vi "Configure Power Measurement Parameter Bandwidth.vi"(6 "Bandwidth":dbl[](array[numeric]) format="%#.9p", 7 "Filter Type (Gauss)":i32(ring) items=["Gauss", "Bandpass"], 8 "error in (no error)":errorcluster, 9 "Array Size (32)":i32=32, 10 "Instance (1)":i32=1, 11 "VISA resource name":refnum<visa-resource-name>) -> (0 "error out":errorcluster, 3 "VISA resource name out":refnum<visa-resource-name>)   [LabVIEW 2020, in "Rohde&Schwarz CMXP GPRF.lvlib"]
doc: "This VI sets is a combination of measurement control settings. The \"Parameter Set List\" contains 32 possibly different parameter sets which you may assign to the individual measurement steps in list mode.\n\nAttributes:\nRSCMXPGPRF_ATTR_POWER_MEASUREMENT_PARAMETER_SET_GAUSS_BW_ALL\nRSCMXPGPRF_ATTR_POWER_MEASUREMENT_PARAMETER_SET_BANDPASS_BW_ALL\n\nRemote-control commands:\nCONFigure:GPRF:MEAS<i>:POWer:PSET:FILTer:GAUSs:BWIDth:ALL\nCONFigure:GPRF:MEAS<i>:POWer:PSET:FILTer:BANDpass:BWIDth:ALL"
uses:
  <instrlib>/Rohde&Schwarz CMXP GPRF/Rohde&Schwarz CMXP GPRF.lvlib
  <instrlib>/Rohde&Schwarz CMXP GPRF/Private/rsidr_core.llb/rsidr_core.lvlib
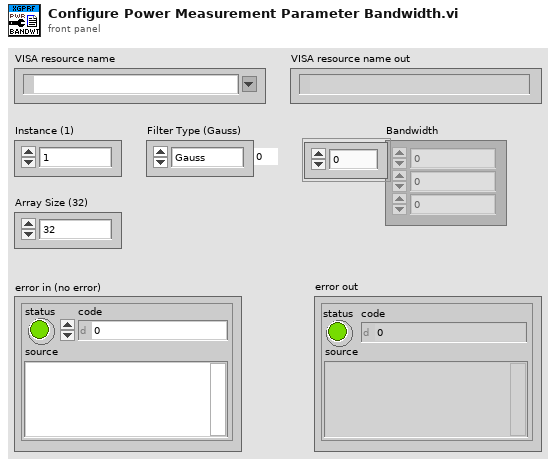
[diagram p1: front panel]
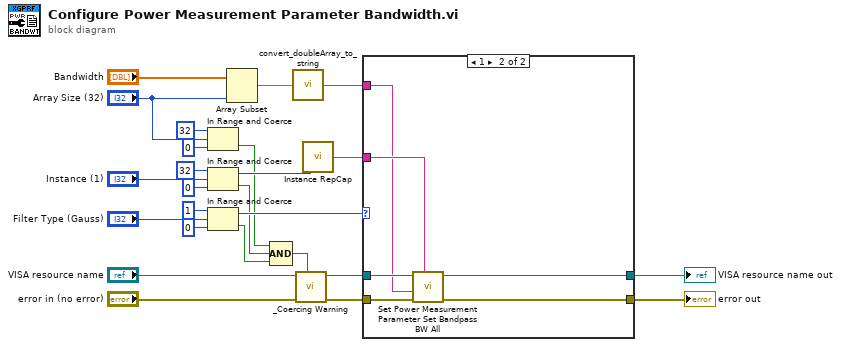
[diagram p0: block diagram]
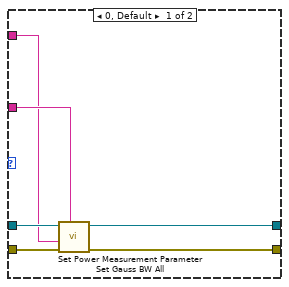
[diagram p2: hidden frame]
diagram:
  n1 = In Range and Coerce(upper limit=32, x="Array Size (32)", lower limit=0) -> (In Range?=w1:bool)  [unwired: 1 out]
  n2 = In Range and Coerce(upper limit=32, x="Instance (1)", lower limit=0) -> (coerced(x)=w14:i32, In Range?=w2:bool)
  n3 = In Range and Coerce(upper limit=1, x="Filter Type (Gauss)", lower limit=0) -> (coerced(x)=w10:i32, In Range?=w3:bool)
  n4 = Array Subset(array="Bandwidth", length="Array Size (32)") -> (w18:dbl[])  [unwired: 1 in]
  n5 = Compound Arithmetic op=AND(w1, w2, w3) -> (w21:bool)
  n6 = call <instrlib>:"convert_doubleArray_to_string.vi"("double array in"=w18) -> ("string out"=w4:string)  [unwired: 4 in]
  n7 = call <instrlib>:"_Coercing Warning.vi"("In Range?"=w21, "error in (no error)"="error in (no error)", "VISA resource name"="VISA resource name") -> ("error out"=w9:errorcluster, "VISA resource name out"=w8:refnum<visa-resource-name>)  [unwired: 7 in]
  n8 = call <instrlib>:"Instance RepCap.vi"("Instance in"=w14) -> ("Instance out"=w5:string)
  n9 = case shown="1" w10 {
    tunnel: w9 -> [w31 w37]
    tunnel: w8 -> [w30 w36]
    tunnel: [w29 w35] -> w7
    tunnel: [w28 w34] -> w6
    tunnel: w5 -> [w27 w33]
    tunnel: w4 -> [w26 w32]
    frame 0, Default {
      n10 = call "Set Power Measurement Parameter Set Gauss BW All"("Repeated Capabilities"=w27, "error in (no error)"=w31, "Power Measurement Parameter Set Gauss BW All ()"=w26, "instrument handle"=w30) -> ("error out"=w29:errorcluster, "instrument handle out"=w28:refnum<visa-resource-name>)  [unwired: 6 in]
    }
    frame 1 {
      n11 = call "Set Power Measurement Parameter Set Bandpass BW All"("Repeated Capabilities"=w33, "error in (no error)"=w37, "Power Measurement Parameter Set Bandpass BW All ()"=w32, "instrument handle"=w36) -> ("error out"=w35:errorcluster, "instrument handle out"=w34:refnum<visa-resource-name>)  [unwired: 6 in]
    }
  }
  "error out" <- w7
  "VISA resource name out" <- w6
